vi "Digital Pattern Wrap Around Array.vi"(9 "Rotations":u16, 11 "x":dbl[](array[numeric])) -> (3 "x":dbl[](array[numeric]))   [LabVIEW 2013, in "Engine Simulation Toolkit System Explorer.lvlib"]
uses:
  Engine Simulation Toolkit System Explorer.lvlib
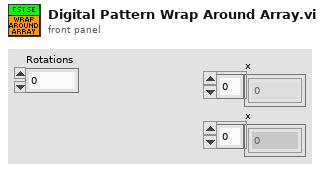
[diagram p1: front panel]
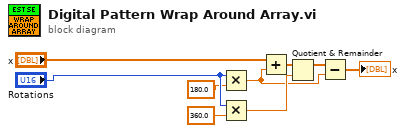
[diagram p0: block diagram]
diagram:
  n1 = Multiply(x="Rotations", y=180.0 ("t")) -> (x*y=w1:dbl)
  n2 = Multiply(x="Rotations", y=360.0 ("t")) -> (x*y=w5:dbl)
  n3 = Add(x="x", y=w1) -> (x+y=w9:dbl[])
  n4 = Quotient & Remainder(x=w9, y=w5) -> (x-y*floor(x/y)=w8:dbl[])  [unwired: 1 out]
  n5 = Subtract(x=w8, y=w1) -> (x-y=→"x":dbl[])
